vi "Parse Bumps + Wheel Drops.vi"(11 "stream in":u8[](array[numeric])) -> (0 "Bumps + Wheel Drops":T1, 3 "stream out":u8[](array[numeric]))   [LabVIEW 2013]
doc: "Read bump and wheeldrop sensors from a UART data stream."
uses:
  Bumps + Wheel Drops.ctl
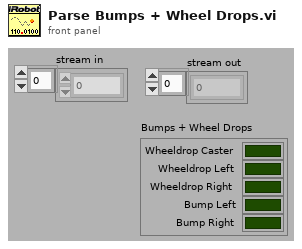
[diagram p1: front panel]
types:
  T1 = typedef "Bumps + Wheel Drops.ctl" = cluster{"Wheeldrop Caster":bool, "Wheeldrop Left":bool, "Wheeldrop Right":bool, "Bump Left":bool, "Bump Right":bool}
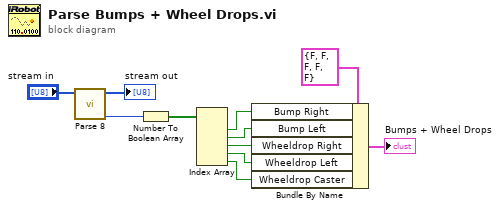
[diagram p0: block diagram]
diagram:
  n1 = call "Parse 8.vi"("stream in"="stream in") -> ("value"=w2:u8, "stream out"=→"stream out":u8[])  [unwired: 9 out]
  n2 = Number To Boolean Array(number=w2) -> (Boolean array=w1:bool[])
  n3 = Index Array(array=w1) -> (element #1=w11:bool, element #2=w8:bool, element #3=w7:bool, element #4=w6:bool, element #5=w5:bool)  [unwired: 5 in]
  n4 = Bundle By Name(cluster=T1 {"Wheeldrop Caster"=FALSE, "Wheeldrop Left"=FALSE, "Wheeldrop Right"=FALSE, "Bump Left"=FALSE, "Bump Right"=FALSE} ("Bumps + Wheel Drops"), "Bump Right"=w11, "Bump Left"=w8, "Wheeldrop Right"=w7, "Wheeldrop Left"=w6, "Wheeldrop Caster"=w5) -> (→"Bumps + Wheel Drops":T1)
